vi "SDSU_SetMux.vi"(6 "muxes index":i32, 7 "fd":i32, 8 "error in (no error)":errorcluster, 9 "muxes in":T1(array[cluster]), 10 "clk":string, 11 "mux":string) -> (0 "error IO":errorcluster, 1 "muxes out":T1(array[cluster]), 2 "response":string)   [LabVIEW 2016]
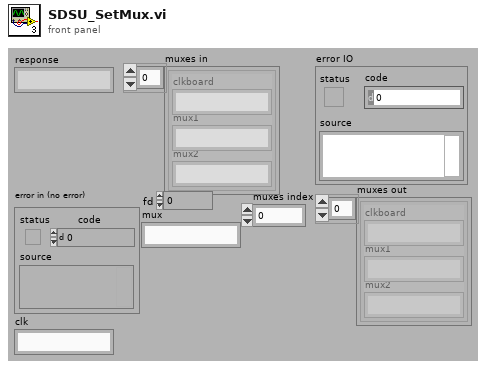
[diagram p1: front panel]
types:
  T1 = cluster{"clkboard":string, "mux1":string, "mux2":string}[]
  T2 = cluster{"clkboard":string, "mux1":string, "mux2":string}
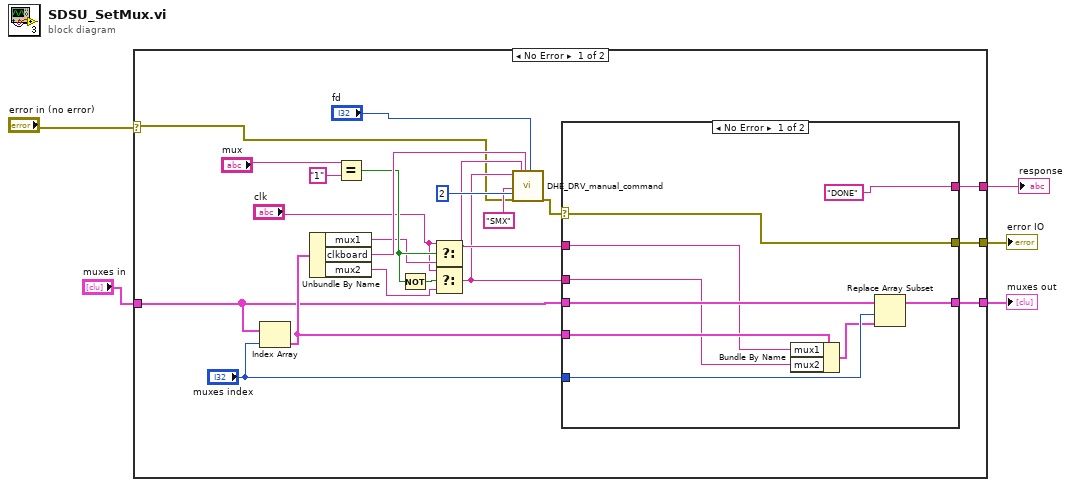
[diagram p0: block diagram]
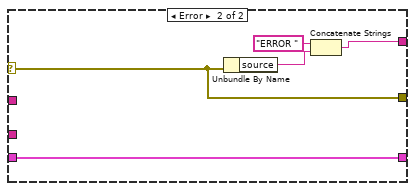
[diagram p2: hidden frame]
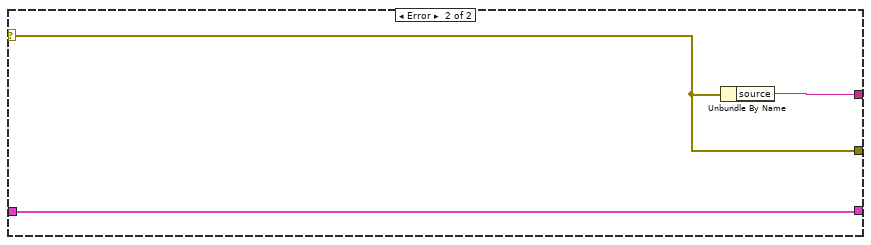
[diagram p3: hidden frame]
diagram:
  n1 = case shown="No Error" "error in (no error)" {
    selector: "error in (no error)" -> [w7 w43]
    tunnel: [w15 w43] -> w5
    tunnel: [w13 w41] -> w4
    tunnel: [w8 w42] -> w3
    tunnel: "muxes in" -> [w6 w41]
    frame No Error {
      n2 = Index Array(array=w6, index="muxes index") -> (element=w11:T2)
      n3 = Unbundle By Name(w11) -> ("mux1"=w19:string, "clkboard"=w23:string, "mux2"=w20:string)
      n4 = Equal?(x="mux", y="1") -> (x = y?=w22:bool)
      n5 = Not(x=w22) -> (.not. x?=w21:bool)
      n6 = Select(t="clk", s=w22, f=w19) -> (s? t:f=w10:string)
      n7 = Select(t="clk", s=w21, f=w20) -> (s? t:f=w9:string)
      n8 = call "DHE_DRV_manual_command.vi"("arg3"=w9, "command"="SMX", "short board_dest"=i16 2, "error in (no error)"=w7, "arg2"=w10, "arg1"=w23, "fd"="fd") -> ("error out"=w18:errorcluster)  [unwired: 2 in, 10 out]
      n9 = case shown="No Error" w18 {
        selector: w18 -> [w35 w39]
        tunnel: w6 -> [w34 w40]
        tunnel: [w35 w39] -> w15
        tunnel: [w32 w40] -> w13
        tunnel: "muxes index" -> [w33 _]
        tunnel: w11 -> [w31 _]
        tunnel: w10 -> [w29 _]
        tunnel: w9 -> [w28 _]
        tunnel: ["DONE" ("mux1") w36] -> w8
        frame No Error {
          n10 = Bundle By Name(cluster=w31, "mux1"=w29, "mux2"=w28) -> (w30:T2)
          n11 = Replace Array Subset(array=w34, new element=w30, index=w33) -> (w32:T1)
        }
        frame Error {
          n12 = Unbundle By Name(w39) -> ("source"=w38:string)
          n13 = Concatenate Strings("ERROR " ("string"), w38) -> (w36:string)
        }
      }
    }
    frame Error {
      n14 = Unbundle By Name(w43) -> ("source"=w42:string)
    }
  }
  "error IO" <- w5
  "muxes out" <- w4
  "response" <- w3
